vi "registerUserEvents.vi"(8 "error in (no error)":errorcluster, 11 "SM1000-control in":T1) -> (0 "error out":errorcluster, 2 "Event Refnum":refnum<event-registration>, 3 "SM1000-control out":T1)   [LabVIEW 2013, in "SLMControl.lvlib" / "SM1000.lvclass"]
doc: "Unregisters the application for 'OnConnect'-events."
uses:
  SM1000.lvclass
  Object-reference.ctl
  SM1000.lvclass/SM1000.ctl
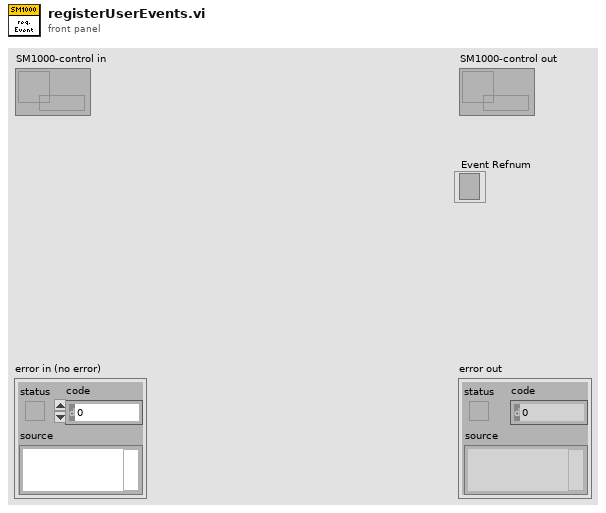
[diagram p1: front panel]
types:
  T1 = typedef "SLMControl.lvlib/SM1000.lvclass/Object-reference.ctl" = refnum<data-value>
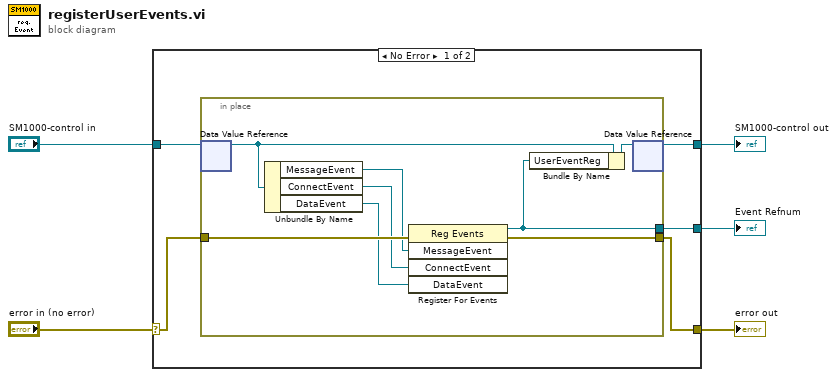
[diagram p0: block diagram]
diagram:
  n1 = case shown="No Error" "error in (no error)" {
    selector: "error in (no error)" -> [w7 w20]
    tunnel: [w8 w20] -> w4
    tunnel: [w9 w19] -> w2
    tunnel: "SM1000-control in" -> [w10 w19]
    tunnel: [w6 _] -> w1
    frame No Error {
      n2 = in-place {
        in-place-border: w7 -> [w16]
        in-place-border: [w17] -> w8
        in-place-border: [w11] -> w6
        n3 = in-place-dvr #1(w10) -> (w18:refnum<class "SM1000.lvclass">)  [unwired: 1 out]
        n4 = Unbundle By Name(w18) -> ("MessageEvent"=w15:refnum<user-event>, "ConnectEvent"=w14:refnum<user-event>, "DataEvent"=w13:refnum<user-event>)
        n5 = register-events(error in=w16, w15, w14, w13) -> (reference out=w11:refnum<event-registration>, error out=w17:errorcluster)  [unwired: 1 in]
        n6 = Bundle By Name(cluster=w18, "UserEventReg"=w11) -> (w12:refnum<class "SM1000.lvclass">)
        n7 = in-place-dvr #1(w12) -> (w9:T1)  [unwired: 1 out]
      }
    }
    frame Error {
    }
  }
  "error out" <- w4
  "SM1000-control out" <- w2
  "Event Refnum" <- w1
